vi "get State.vi"(11 "Control State in":refnum<class "Control State.lvclass">) -> (0 "Thrust":T1=enum."Pressed", 1 "Special Function":T1=enum."Pressed", 2 "Primary Weapon":T1=enum."Pressed", 4 "Rotate Clockwise":T1=enum."Pressed", 6 "Rotate Counter Clockwise":T1=enum."Pressed")   [LabVIEW 2015, in "Control State.lvclass"]
uses:
  Control State.lvclass
  Button State.ctl
  Control State.lvclass/Control State.ctl
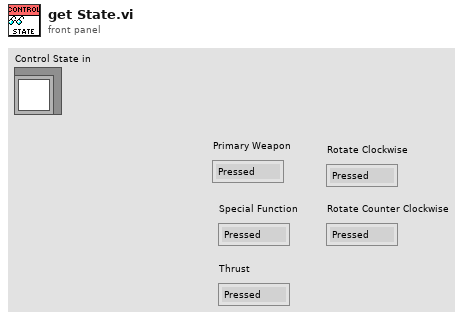
[diagram p1: front panel]
types:
  T1 = typedef "Control State.lvclass/Button State.ctl" = enum16{"Undefined", "Pressed", "Released", "Held", "Not Held"}
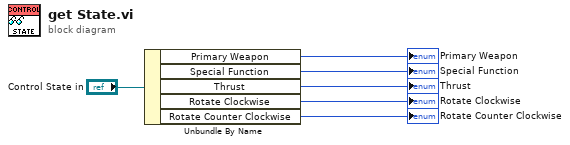
[diagram p0: block diagram]
diagram:
  n1 = Unbundle By Name("Control State in") -> ("Primary Weapon"=→"Primary Weapon":T1, "Special Function"=→"Special Function":T1, "Thrust"=→"Thrust":T1, "Rotate Clockwise"=→"Rotate Clockwise":T1, "Rotate Counter Clockwise"=→"Rotate Counter Clockwise":T1)
